vi "#111_MAV_MSG_TIMESYNC_ENCODE.vi"(10 "packet_sequence_in":u8, 11 "TIMESYNC":T1={"self"={"system_id"=255, "component_id"=190}, "target_system"=1, "target_component"=1, "tc1 (ns)"=0, "ts1 (ns)"=0}) -> (2 "packet_sequence_out":u8, 3 "mavlink_buffer_out":u8[](array[numeric]))   [LabVIEW 2023]
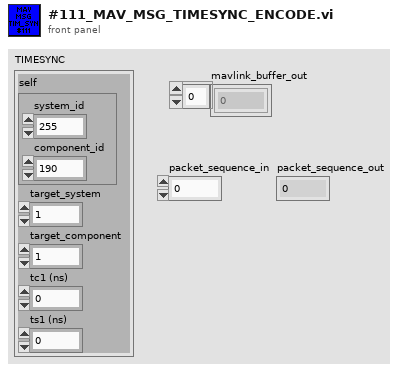
[diagram p1: front panel]
types:
  T1 = cluster{"self":cluster{"system_id":u8, "component_id":u8}, "target_system":u8, "target_component":u8, "tc1 (ns)":i64, "ts1 (ns)":i64}
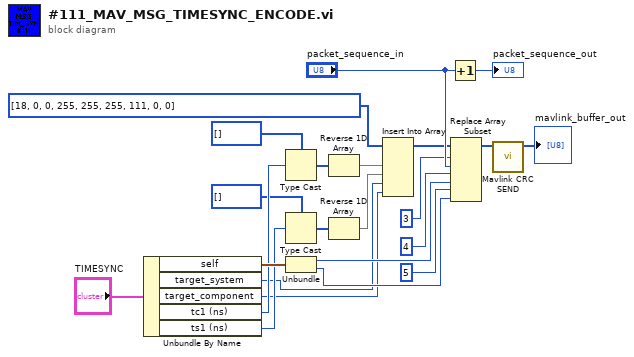
[diagram p0: block diagram]
diagram:
  n1 = Unbundle By Name("TIMESYNC") -> ("self"=w14:cluster{"system_id":u8, "component_id":u8}, "target_system"=w3:u8, "target_component"=w2:u8, "tc1 (ns)"=w9:i64, "ts1 (ns)"=w6:i64)
  n2 = Type Cast(type=u8[] [] ("index"), x=w9) -> (*(type *) &x=w10:u8[])
  n3 = Type Cast(type=u8[] [] ("index"), x=w6) -> (*(type *) &x=w7:u8[])
  n4 = Unbundle(w14) -> ("system_id"=w13:u8, "component_id"=w12:u8)
  n5 = Reverse 1D Array(array=w10) -> (reversed array=w5:u8[])
  n6 = Reverse 1D Array(array=w7) -> (reversed array=w4:u8[])
  n7 = Insert Into Array(array=u8[] [18, 0, 0, 255, 255, 255, 111, 0, 0], new element #1=w5, new element #2=w4, new element #3=w3, new element #4=w2) -> (w21:u8[])  [unwired: 1 in]
  n8 = Increment(x="packet_sequence_in") -> (x+1=→"packet_sequence_out":u8)
  n9 = Replace Array Subset(array=w21, new element #1="packet_sequence_in", index #1=3 ("index"), new element #2=w13, index #2=4 ("index"), new element #3=w12, index #3=5 ("index")) -> (w19:u8[])
  n10 = call "Mavlink CRC SEND.vi"("Byte In"=w19) -> ("Output Byte"=→"mavlink_buffer_out":u8[])  [unwired: 10 in]
